vi "4Pi DCM - Wait New Frame.vi"(0 "Camera Notifier Name":string, 13 "Wait No. (1)":u32=1) -> (4 "Camera Notifier Name (Dup)":string)   [LabVIEW 2016]
uses:
  Device Library/Cameras/Hamamatsu/Orca Flash/Orca Flash Controls/Orca Flash Actions.ctl
  Device Library/Cameras/Camera Controls/Camera IMAQ Key Info.ctl
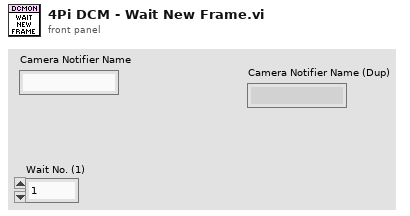
[diagram p1: front panel]
types:
  T1 = typedef "Camera IMAQ Key Info.ctl" = cluster{"Frame":u32, "Sensor Height":i32, "Sensor Width":i32, "ROI Height":i32, "ROI Width":i32, "ROI Enable?":bool, "Bit per Pixel":u8}
  T2 = typedef "Orca Flash Actions.ctl" = enum16{"IDLE", "PREVIEW", "RECORD", "Send Trigger", "SOFT TRIGGER", "Record Settings", "SETPARAM", "GETPARAM", "SETROI", "GETROI", "PROGRESSIVE MODE", "AREA MODE", "STATUS", "QUIT"}
  T3 = typedef "IMAQ Image.ctl" = refnum<image>
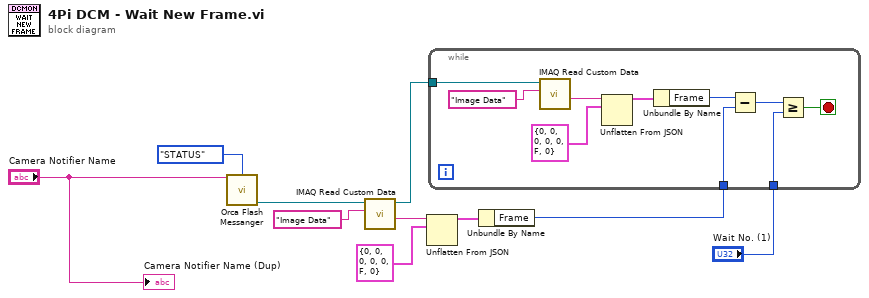
[diagram p0: block diagram]
diagram:
  n1 = call "Orca Flash Messanger.vi"("Notifier Name"="Camera Notifier Name", "Camera Actions"=Orca_Flash_Actions."STATUS") -> ("Image Ref"=w5:T3)  [unwired: 9 in, 4 out]
  n2 = call "IMAQ Read Custom Data"("Key"="Image Data", "Image"=w5) -> ("Custom Data Out"=w7:string, "Image (duplicate)"=w4:T3)  [unwired: 7 in, 1 out]
  n3 = Unflatten From JSON(JSON string=w7, type and defaults=T1 {"Frame"=0, "Sensor Height"=0, "Sensor Width"=0, "ROI Height"=0, "ROI Width"=0, "ROI Enable?"=FALSE, "Bit per Pixel"=0} ("Camera IMAQ Key Info")) -> (value=w9:T1)  [unwired: 5 in, 1 out]
  n4 = Unbundle By Name(w9) -> ("Frame"=w3:u32)
  n5 = while {
    tunnel: w4 -> [w16]
    tunnel: w3 -> [w14]
    tunnel: "Wait No. (1)" -> [w11]
    stop <- w12 stop-if-true
    n6 = call "IMAQ Read Custom Data"("Key"="Image Data", "Image"=w16) -> ("Custom Data Out"=w18:string)  [unwired: 7 in, 2 out]
    n7 = Unflatten From JSON(JSON string=w18, type and defaults=T1 {"Frame"=0, "Sensor Height"=0, "Sensor Width"=0, "ROI Height"=0, "ROI Width"=0, "ROI Enable?"=FALSE, "Bit per Pixel"=0} ("Camera IMAQ Key Info")) -> (value=w20:T1)  [unwired: 5 in, 1 out]
    n8 = Unbundle By Name(w20) -> ("Frame"=w15:u32)
    n9 = Subtract(x=w15, y=w14) -> (x-y=w13:u32)
    n10 = Greater Or Equal?(x=w13, y=w11) -> (x >= y?=w12:bool)
  }
  "Camera Notifier Name (Dup)" <- "Camera Notifier Name"
